vi "load control values from file.vi"(8 "error in (no error)":errorcluster, 10 "datalog path (use dialog)":path, 11 "VI ref":refnum<vi>) -> (0 "error out":errorcluster)   [LabVIEW 2021]
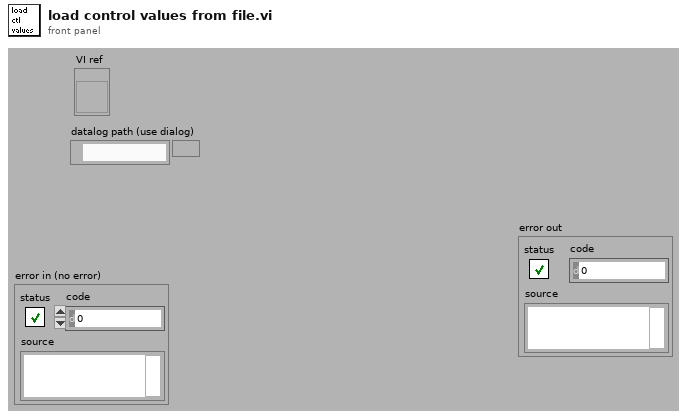
[diagram p1: front panel]
types:
  T1 = enum16{"open", "replace", "create", "open or create", "replace or create", "replace or create with confirmation"}
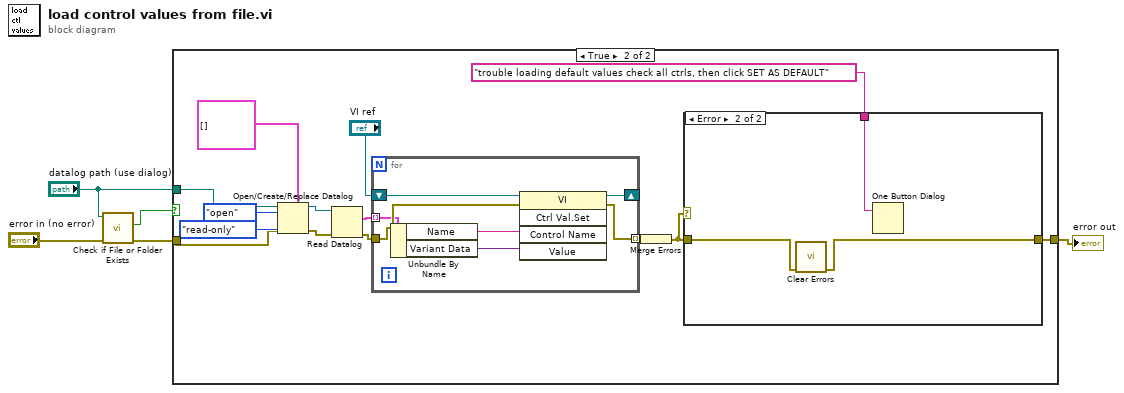
[diagram p0: block diagram]
diagram:
  n1 = call <vilib>:"Check if File or Folder Exists.vi"("error in (no error)"="error in (no error)", "path"="datalog path (use dialog)") -> ("error out"=w3:errorcluster, "file or folder exists?"=w1:bool)  [unwired: 7 in, 1 out]
  n2 = case shown="True" w1 {
    tunnel: [w6 w11] -> w5
    tunnel: "datalog path (use dialog)" -> [_ w9]
    tunnel: w3 -> [w6 w8]
    frame False {
    }
    frame True {
      n3 = Open/Create/Replace Datalog(5:cluster{"Name":string, "Variant Data":variant}[] [] ("Control Value:Get All [Variant]"), 8:w8, 9:enum16{"read/write", "read-only", "write-only"}."read-only" ("access (0:read/write)"), 10:T1."open" ("operation (0:open)"), 11:w9) -> (0:w18:errorcluster, 3:w17:refnum<k1>)  [unwired: 1 in, 1 out]
      n4 = Read Datalog(4:w18, 7:w17) -> (0:w15:errorcluster, 2:w16:cluster{"Name":string, "Variant Data":variant}[])  [unwired: 1 in, 1 out]
      n5 = for {
        tunnel: w16 -> [w29] mode=indexing
        shift-right: [w25] -> _
        shift-left: "VI ref" -> [w31]
        tunnel: w15 -> [w30]
        tunnel: [w26] -> w12 mode=indexing
        n6 = Unbundle By Name(w29) -> ("Name"=w28:string, "Variant Data"=w27:variant)
        n7 = invoke class="VI" method="Ctrl Val.Set"(reference=w31, error in=w30, "Control Name"=w28, "Value"=w27) -> (reference out=w25:refnum<vi>, error out=w26:errorcluster)  [unwired: 1 in, 3 out]
      }
      n8 = Merge Errors(w12) -> (w7:errorcluster)
      n9 = case shown="Error" w7 {
        tunnel: w7 -> [w21 w23]
        tunnel: [w21 w22] -> w11
        tunnel: "trouble loading default values check all ctrls, then click SET AS DEFAULT" ("message") -> [_ w24]
        frame No Error {
        }
        frame Error {
          n10 = call <vilib>:"Clear Errors.vi"("error in (no error)"=w23) -> ("error out"=w22:errorcluster)  [unwired: 5 in, 1 out]
          n11 = One Button Dialog(message=w24) -> ()  [unwired: 1 in, 1 out]
        }
      }
    }
  }
  "error out" <- w5
